vi "Untitled 1.vi"() -> ()   [LabVIEW 2017]
uses:
  <vilib>/addons/database/Connection.llb/DB Tools Open Connec (Path).vi
  <vilib>/addons/database/NI_Database_API.lvlib
panel:
  out "ISO-8601 UTC Formatted DateTime String":string
  out "error out 2":errorcluster
  in  "error in":errorcluster
  out "error out":errorcluster
  in  "Boolean":bool
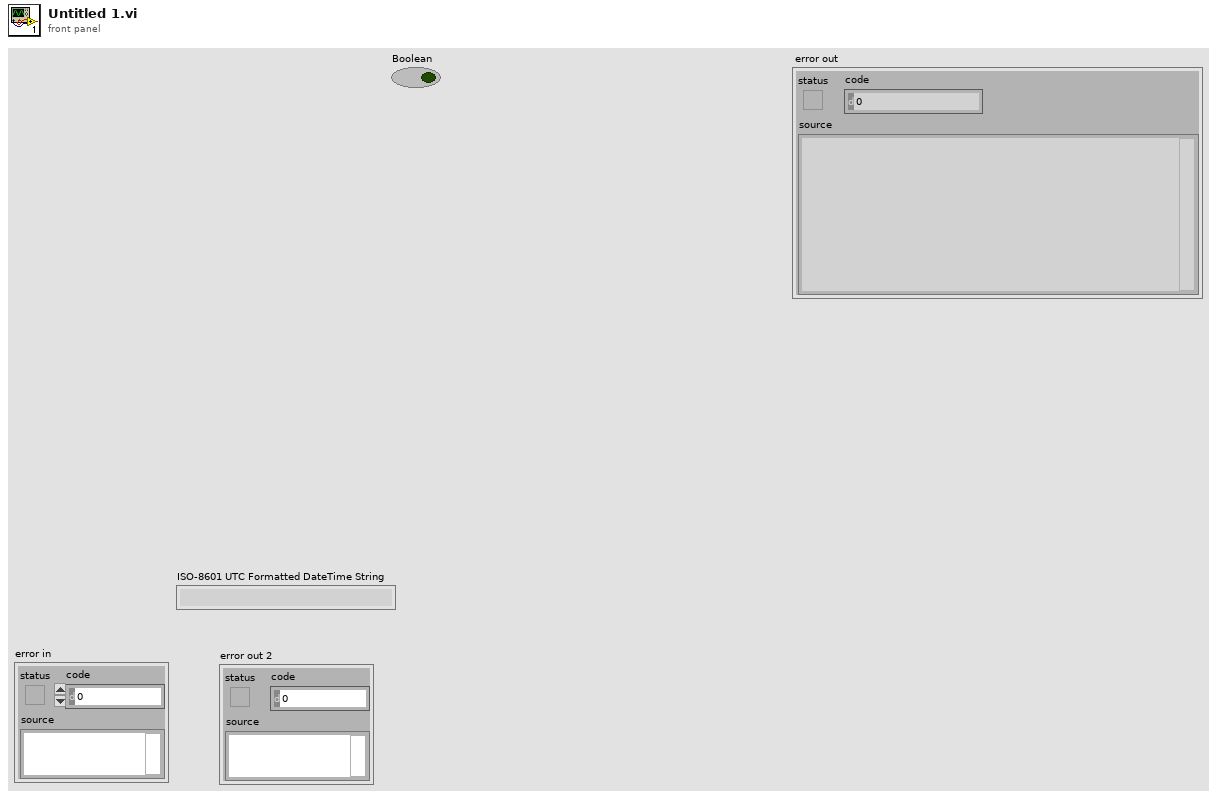
[diagram p1: front panel]
types:
  T1 = typedef "NI_Database_API.lvlib/Conn ObjectReference.ctl" = refnum<k1>
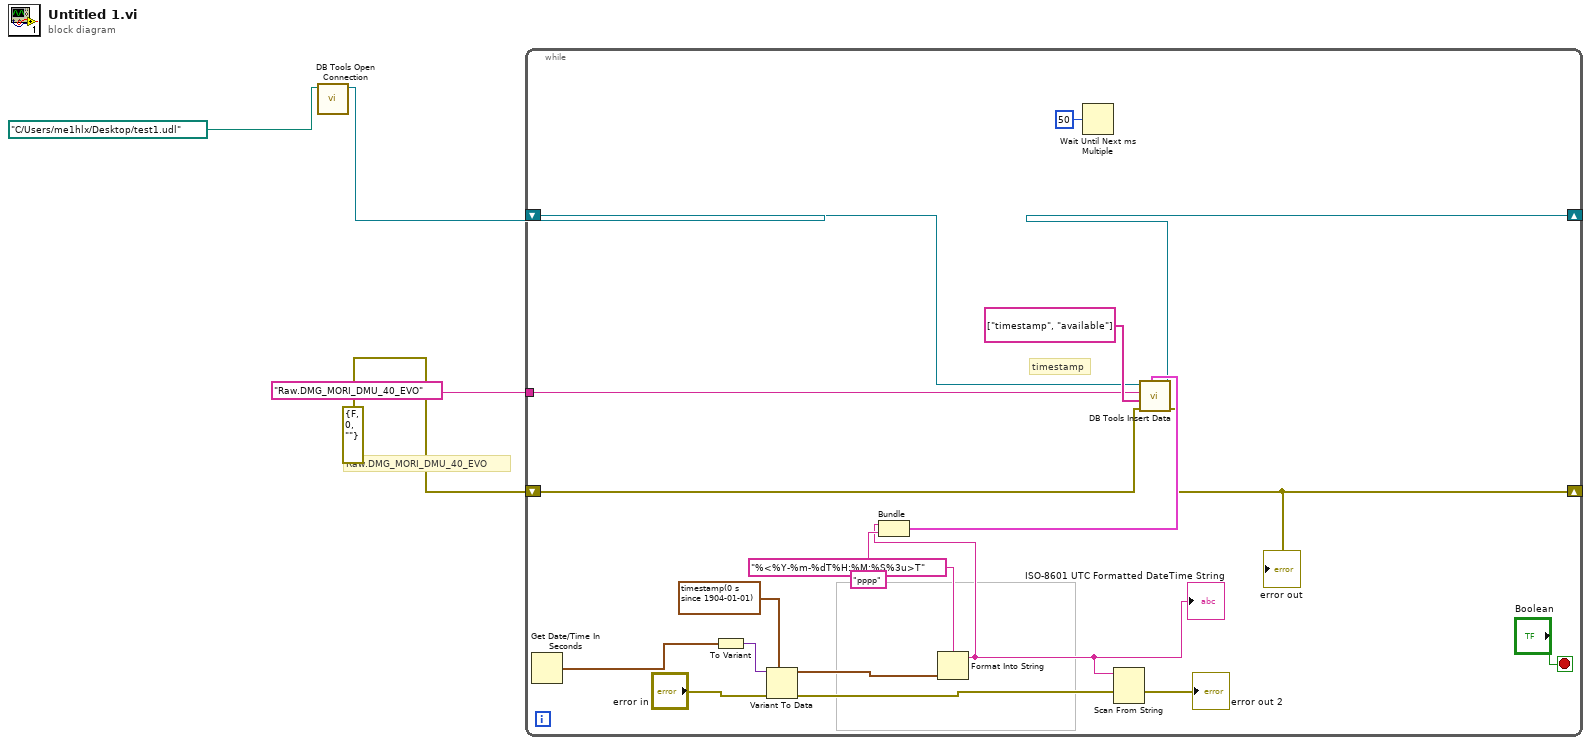
[diagram p0: block diagram]
diagram:
  # "Raw.DMG_MORI_DMU_40_EVO"
  n1 = call-poly <vilib>:"DB Tools Open Connection.vi"("connection information"=path "C:/Users/me1hlx/Desktop/test1.udl") -> ("connection reference"=w3:T1)  [unwired: 7 in, 1 out]
  n2 = while {
    shift-right: [w19] -> _
    shift-left: w3 -> [w20]
    tunnel: "Raw.DMG_MORI_DMU_40_EVO" -> [w21]
    shift-right: [w17] -> _
    shift-left: errorcluster {"status"=FALSE, "code"=0, "source"=""} ("error in (no error)") -> [w18]
    stop <- "Boolean" stop-if-true
    # "timestamp"
    n3 = Get Date/Time In Seconds() -> (seconds since 1Jan1904=w12:timestamp)
    n4 = To Variant(anything=w12) -> (Variant=w7:variant)
    n5 = Variant To Data(error in="error in", type=timestamp(0 s since 1904-01-01) ("time stamp"), Variant=w7) -> (data=w11:timestamp, error out=w9:errorcluster)
    n6 = Format Into String(format string="%<%Y-%m-%dT%H:%M:%S%3u>T", w11) -> (resulting string=w13:string)  [unwired: 2 in, 1 out]
    "ISO-8601 UTC Formatted DateTime String" <- w13
    n7 = Bundle(w13, "pppp") -> (w22:cluster{string, string})  [unwired: 1 in]
    n8 = Wait Until Next ms Multiple(millisecond multiple=u32 50) -> ()  [unwired: 1 out]
    n9 = Scan From String(input string=w13, error in=w9) -> (error out=→"error out 2":errorcluster)  [unwired: 4 in, 2 out]
    n10 = call <vilib>:"DB Tools Insert Data.vi"("data"=w22, "error in (no error)"=w18, "columns"=string[] ["timestamp", "available"], "table"=w21, "connection reference"=w20) -> ("error out"=w17:errorcluster, "connection reference out"=w19:T1)  [unwired: 5 in]
    "error out" <- w17
  }
